vi "DelayedRX.vi"(9 "Module ID":i32=-1, 10 "milliseconds to wait":u32) -> ()   [LabVIEW 2015, in "Serializer.lvlib"]
uses:
  Serializer.lvlib
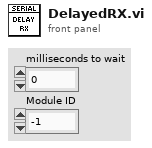
[diagram p1: front panel]
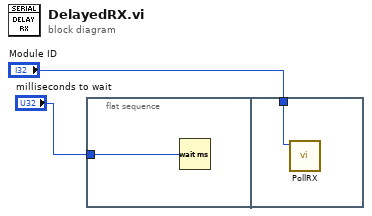
[diagram p0: block diagram]
diagram:
  n1 = flat-sequence {
    tunnel: "milliseconds to wait" -> [w3]
    tunnel: "Module ID" -> [w4]
    frame #0 {
      n2 = Wait (ms)(milliseconds to wait=w3) -> ()  [unwired: 1 out]
    }
    frame #1 {
      n3 = call "PollRX.vi"("Module ID"=w4) -> ()  [unwired: 10 in, 1 out]
    }
  }
